vi "r11.vi"() -> ()   [LabVIEW 2019]
panel:
  out "error out":errorcluster
  in  "error in (no error)":errorcluster
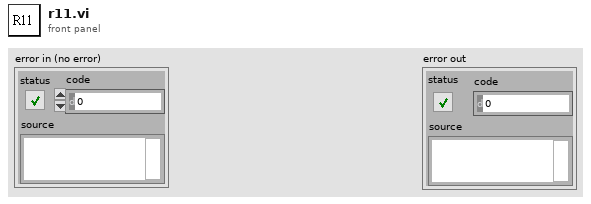
[diagram p1: front panel]
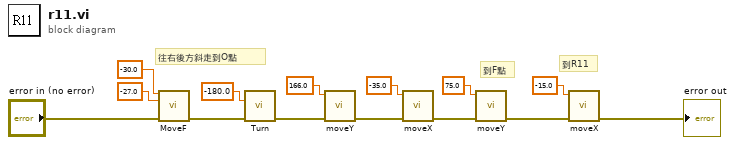
[diagram p0: block diagram]
diagram:
  # "到R11"
  # "到F點"
  # "往右後方斜走到O點"
  n1 = call "MoveF.vi"("X"=-30.0, "Y"=-27.0, "error in (no error)"="error in (no error)") -> ("error out"=w11:errorcluster)  [unwired: 12 in]
  n2 = call "Turn.vi"("角度"=-180.0, "error in (no error)"=w11) -> ("error out"=w10:errorcluster)  [unwired: 13 in]
  n3 = call "moveY.vi"("error in (no error)"=w10, "Y"=166.0) -> ("error out"=w8:errorcluster)  [unwired: 9 in]
  n4 = call "moveX.vi"("error in (no error)"=w8, "X"=-35.0) -> ("error out"=w6:errorcluster)  [unwired: 9 in]
  n5 = call "moveY.vi"("error in (no error)"=w6, "Y"=75.0) -> ("error out"=w3:errorcluster)  [unwired: 9 in]
  n6 = call "moveX.vi"("error in (no error)"=w3, "X"=-15.0) -> ("error out"=→"error out":errorcluster)  [unwired: 9 in]
